vi "PH_ImageOperator.Show Image.vi"(0 "i ref in":refnum<vi>, 5 "error out":errorcluster) -> (14 "i ref out":refnum<vi>, 19 "error out":errorcluster)   [LabVIEW 2014, in "PH_ImageOperator.lvlib"]
doc: "This VI sets copies the operator image, sets additional information and plots it at the GUI element."
uses:
  PH_ImageOperator.lvlib
  PH_Basics/PH_Image_Common/PH_Image_Common.lvlib
  PH_Basics/PH_Img_BaseClass/PH_Img_BaseClass.lvlib
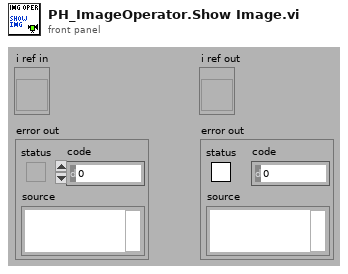
[diagram p1: front panel]
types:
  T1 = typedef "PH_ImageOperator.lvlib/PH_ImageOperator.i attribute.ctl" = cluster{"GUI Refs":cluster{"Delete":refnum<vi>, "Calibration status":refnum<vi>, "BI subtracted":refnum<vi>, "calc Energy":refnum<vi>, "Energy: expected value":refnum<vi>, "Energy: Tolerance":refnum<vi>, "Energy calculated":refnum<vi>, "Energy":refnum<vi>, "calc Beam Anal":refnum<vi>, "Maj Diam 1/esquare":refnum<vi>, "Min Diam 1/esquare":refnum<vi>, "Azi Angle":refnum<vi>, "Min/Maj Diam esquare":refnum<vi>, "Beam analysed":refnum<vi>, "CoG - x":refnum<vi>, "CoG - y":refnum<vi>, "BA: Method":refnum<vi>, "BA: Steps":refnum<vi>, "BA: Factor":refnum<vi>, "calc Traces":refnum<vi>, "Traces: Fit Gauss":refnum<vi>, "Traces calculated":refnum<vi>, "Maj FWHM":refnum<vi>, "Min FWHM":refnum<vi>, "Major Trace":refnum<vi>, "Minor Trace":refnum<vi>, "Maj Fit Order":refnum<vi>, "Min Fit Order":refnum<vi>, "Position calculated":refnum<vi>, "Position":refnum<vi>, "Type":refnum<vi>, "Center":refnum<vi>, "exp - X":refnum<vi>, "exp - Y":refnum<vi>, "Tolerance":refnum<vi>, "f":refnum<vi>, "M":refnum<vi>, "D":refnum<vi>, "q":refnum<vi>, "Dummy Method":refnum<vi>, "Dummy Type":refnum<vi>, "Global On":refnum<vi>, "Traces: No offset":refnum<vi>, "Maj 99%":refnum<vi>, "Min 99%":refnum<vi>, "GUI FF Image":refnum<vi>, "calc Fill Factor":refnum<vi>, "FF calculated":refnum<vi>, "Fill Factor: Filter?":refnum<vi>, "FF: Damage Threshold":refnum<vi>, "FF: Threshold":refnum<vi>, "FF: max allow. Energy":refnum<vi>, "FF: Fillfactor":refnum<vi>, "Calibration data":refnum<vi>}, "List of GUIs":string[], "Calibration":cluster{"Status":T2, "Calibration data":T3, "Calibration Data File":path}, "Final Image":cluster{"BI Subtraction Failure":bool}, "Energy":cluster{"on":bool, "expected value [mJ]":dbl, "Tolerance [%]":dbl, "State":T2, "Energy [mJ]":dbl, "Unit":string, "calculated @":timestamp}, "Beam Analysis":cluster{"on":bool, "Data":T4, "Method":bool, "Steps":i32, "Factor":i32, "ROI":cluster{"Left":i32, "Top":i32, "Right":i32, "Bottom":i32}, "analysed @":timestamp}, "Trace Analysis":cluster{"on":bool, "Fit on":bool, "Maj FWHM":dbl, "Min FWHM":dbl, "Maj Fit Order":i32, "Min Fit Order":i32, "No Offset":bool, "Maj 99%":dbl, "Min 99%":dbl, "Traces":cluster{"XScaleName":string, "Y Scale Minimum":sgl, "Y Scale Maximum":sgl, "X Scale Minimum":sgl, "X Scale Maximum":sgl, "Traces":cluster{"Index":sgl[], "Trace":dbl[]}[]}[], "analysed @":timestamp}, "Position Analysis":cluster{"on":bool, "exp - X":i32, "exp - Y":i32, "focal length [mm]":dbl, "Magnification":dbl, "Delta":dbl, "Theta":dbl, "Tolerance":dbl, "Type":bool, "analysed @":timestamp}, "Fill Factor":cluster{"on":bool, "Filter on?":bool, "Threshold":dbl, "Damage Threshold [J/cm²]":dbl, "Fillfactor":dbl, "Max. allowed Energy [J]":dbl, "calculated @":timestamp}, "Statistician Service ID":i32, "Images":cluster{"Background":T5, "OP":T5, "GUI":T5, "BA: ROI":T5, "Trace: Turn":T5, "FF: Main":T5, "FF: Help":T5, "PSDB: BG":T5, "PSDB: OP":T5, "PSDB: FF":T5}}
  T2 = typedef "PH_StatusHandler.lvlib/PH_StatusHandler.Status.ctl" = i16
  T3 = typedef "PH_ImageCalibrator.lvlib/PH_ImageCalibrator.Calibration Data.ctl" = cluster{"Date":string, "Time":string, "Cam Settings":cluster{"Cam ID":string, "Gain":dbl, "Brightness":dbl, "Shutter":dbl, "Cam Error":bool, "Mode":i32}, "Background Image":cluster{"Image":dbl[][], "Image Error":bool}, "Linear Calibration":cluster{"Calibration Factor":dbl, "not mm or mrad":bool}, "Energy Calibration":cluster{"Calibration Factor":dbl, "no mJ":bool}}
  T4 = typedef "PH_ImageOperator.lvlib/PH_ImageOperator.Beam Analysis Data.ctl" = cluster{"CoG-x":sgl, "CoG-y":sgl, "Maj Dim":dbl, "Min Dim":dbl, "Ellipticity":dbl, "Azimuth Angle [rad]":dbl, "Azi Angle rel to Maj?":bool}
  T5 = typedef "IMAQ Image.ctl" = refnum<image>
  T6 = typedef "PH_Img_BaseClass.lvlib/PH_Img_BaseClass.i attribute.ctl" = cluster{"GUI Refs":T7, "Timeout Image [ms]":i32, "Default Periodic Period [ms]":i32, "Camera":cluster{"Instancename":string, "Notifier":refnum<notifier>}, "Palette":T8, "Cam Settings":cluster{"Cam ID":string, "Gain":dbl, "Brightness":dbl, "Shutter":dbl, "Cam Info Failure":bool, "Mode":i32}}
  T7 = typedef "PH_Img_BaseClass.lvlib/PH_Img_BaseClass.GUI Refs.ctl" = cluster{"Timeout":refnum<vi>, "Image":refnum<vi>, "Palette":refnum<vi>, "Timeout Set":refnum<vi>}
  T8 = typedef "PH_Img_BaseClass.lvlib/PH_Img_BaseClass.Palette.ctl" = i32
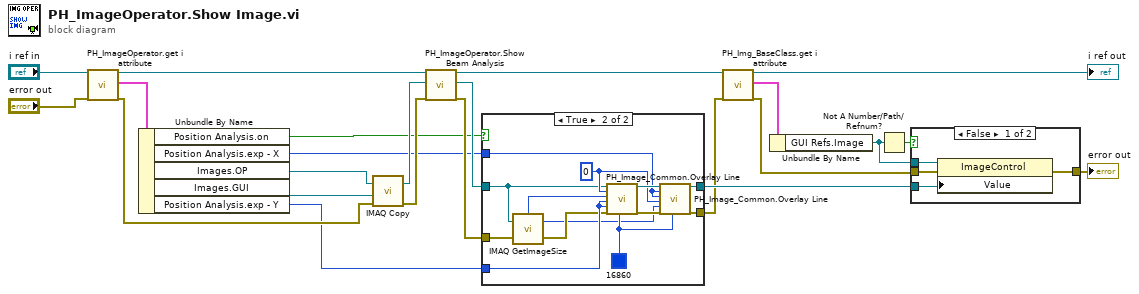
[diagram p0: block diagram]
diagram:
  n1 = call "PH_ImageOperator.get i attribute.vi"("i ref in"="i ref in", "error in (no error)"="error out") -> ("i ref out"=w18:refnum<vi>, "i attribute"=w22:T1, "error out"=w9:errorcluster)  [unwired: 15 in]
  n2 = Unbundle By Name(w22) -> ("Position Analysis.on"=w10:bool, "Position Analysis.exp - X"=w11:i32, "Images.OP"=w7:T5, "Images.GUI"=w6:T5, "Position Analysis.exp - Y"=w8:i32)
  n3 = call "IMAQ Copy"("error in (no error)"=w9, "Image Dst"=w6, "Image Src"=w7) -> ("error out"=w12:errorcluster, "Image Dst Out"=w16:T5)  [unwired: 3 in]
  n4 = call "PH_ImageOperator.Show Beam Analysis.vi"("i ref in"=w18, "GUI Image In"=w16, "error in (no error)"=w12) -> ("i ref out"=w17:refnum<vi>, "GUI Image Out"=w14:T5, "error out"=w15:errorcluster)  [unwired: 14 in]
  n5 = case shown="True" w10 {
    tunnel: w15 -> [w24 w29]
    tunnel: w14 -> [w25 w30]
    tunnel: [w24 w35] -> w3
    tunnel: [w25 w34] -> w13
    tunnel: w11 -> [_ w32]
    tunnel: w8 -> [_ w31]
    frame False {
    }
    frame True {
      w33 = 0 ("Start y")
      w36 = u32 16860 ("Color (red)")
      n6 = call "IMAQ GetImageSize"("Image"=w30, "error in (no error)"=w29) -> ("Y Resolution"=w26:i32, "X Resolution"=w27:i32, "error out"=w28:errorcluster)  [unwired: 2 in]
      n7 = call "PH_Image_Common.Overlay Line.vi"("Image"=w30, "Start x"=w33, "End x"=w27, "Start y"=w31, "End y"=w31, "error in (no error)"=w28, "Color (red)"=w36) -> ("Image Out"=w38:T5, "error out"=w37:errorcluster)  [unwired: 11 in]
      n8 = call "PH_Image_Common.Overlay Line.vi"("Image"=w38, "Start x"=w32, "End x"=w32, "Start y"=w33, "End y"=w26, "error in (no error)"=w37, "Color (red)"=w36) -> ("Image Out"=w34:T5, "error out"=w35:errorcluster)  [unwired: 11 in]
    }
  }
  n9 = call "PH_Img_BaseClass.get i attribute.vi"("i ref in"=w17, "error in (no error)"=w3) -> ("i ref out"=→"i ref out":refnum<vi>, "i attribute"=w2:T6, "error out"=w4:errorcluster)  [unwired: 15 in]
  n10 = Unbundle By Name(w2) -> ("GUI Refs.Image"=w1:refnum<vi>)
  n11 = Not A Number/Path/Refnum?(number/path/refnum=w1) -> (NaN/Path/Refnum?=w19:bool)
  n12 = case shown="False" w19 {
    tunnel: w1 -> [w42 _]
    tunnel: [w41 w43] -> w20
    tunnel: w13 -> [w40 _]
    tunnel: w4 -> [w39 w43]
    frame False {
      n13 = property class="ImageControl"(reference=w42, error in=w39, "Value"=w40) -> (error out=w41:errorcluster)  [unwired: 1 out]
    }
    frame True {
    }
  }
  "error out" <- w20
